vi "TAI_Motor.vi"(2 "Normal Output":dbl, 3 "Actuator Name":string) -> (0 "Interlock Output":dbl, 1 "Testing This Actuator":bool)   [LabVIEW 2019]
doc: "This VI functions as an interlock, allowing operators to bypass the control logic for each actuator and test it using basic commands. This VI supports both floating point and boolean outputs. It requires integration with global variables storing the test signal and the operator's actuator selection. It is intended to integrate with the standard FRC 4265 control architecture."
uses:
  dsdata.vi
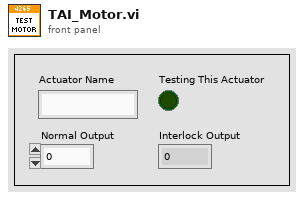
[diagram p1: front panel]
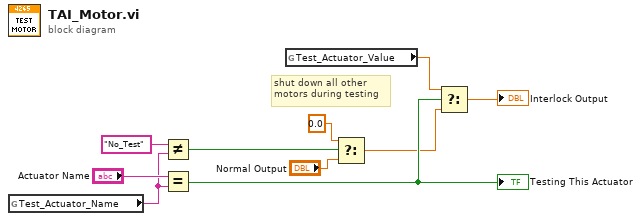
[diagram p0: block diagram]
diagram:
  # "shut down all other\nmotors during testing"
  n1 = global read "dsdata.vi" "Test_Actuator_Name"() -> (w1:string)
  n2 = Not Equal?(x="No_Test", y=w1) -> (x != y?=w2:bool)
  n3 = Equal?(x="Actuator Name", y=w1) -> (x = y?=w8:bool)
  "Testing This Actuator" <- w8
  n4 = global read "dsdata.vi" "Test_Actuator_Value"() -> (w9:dbl)
  n5 = Select(t=0.0, s=w2, f="Normal Output") -> (s? t:f=w3:dbl)
  n6 = Select(t=w9, s=w8, f=w3) -> (s? t:f=→"Interlock Output":dbl)
